vi "Configure Modulation (AM).vi"(4 "Modulation Waveform (0: Sine)":u16(ring) items=["Sine", "Square", "Triangle", "UpRamp", "DnRamp", "Noise", "Arb"], 5 "Channel (1:Channel 1)":i32(ring)=1 items=["Channel 1"=1, "Channel 2"=2], 6 "Modulation Frequency (100 Hz)":dbl=100.0, 7 "Enable Amplitude Modulation (T:Enable)":bool=TRUE, 8 "error in (no error)":errorcluster, 9 "Modulation Depth (0.0 %)":dbl min=0.0 max=120.0 format="%.1f", 10 "AM Source (0: Internal)":u16(ring) items=["Internal", "External"], 11 "VISA resource name":refnum<visa-resource-name>) -> (0 "error out":errorcluster, 3 "VISA resource name out":refnum<visa-resource-name>)   [LabVIEW 2015, in "SDG X Series.lvlib"]
doc: "Configures and enables amplitude modulation (AM). In AM, the amplitude of the carrier is varied by the amplitude of the modulating waveform. \n\n<B>Note:</B> The carrier waveform shape and parameters are set by the Configure Standard Waveform VI."
uses:
  <instrlib>/SDG X Series/SDG X Series.lvlib
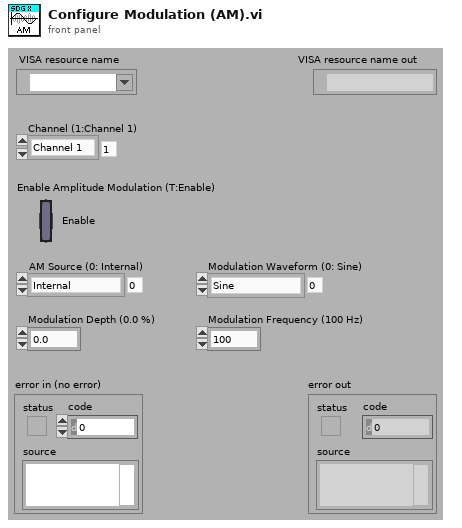
[diagram p1: front panel]
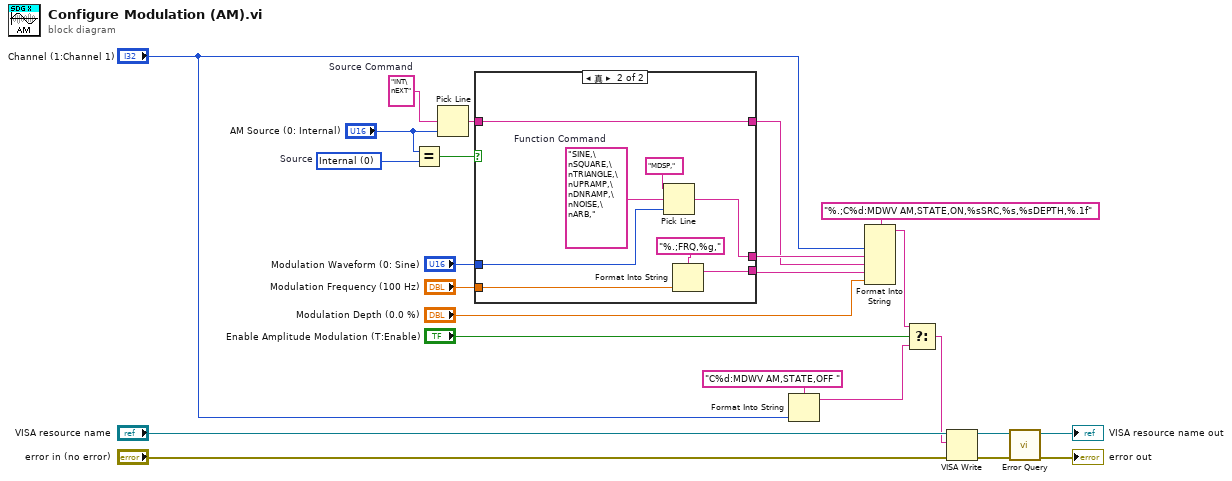
[diagram p0: block diagram]
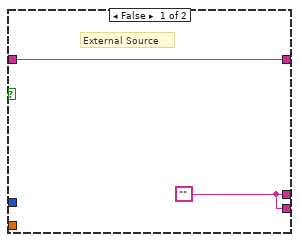
[diagram p2: hidden frame]
diagram:
  w18 = u16 0 items=["Internal", "External"]  # Source
  w19 = "INT\nEXT"  # Source Command
  n1 = Equal?(x="AM Source (0: Internal)", y=w18) -> (x = y?=w17:bool)
  n2 = Pick Line(multi-line string=w19, line index="AM Source (0: Internal)") -> (output string=w16:string)  [unwired: 1 in]
  n3 = case shown="真" w17 {
    tunnel: w16 -> [w26 w32]
    tunnel: "Modulation Waveform (0: Sine)" -> [_ w33]
    tunnel: "Modulation Frequency (100 Hz)" -> [_ w29]
    tunnel: [w26 w32] -> w13
    tunnel: [w25 w30] -> w14
    tunnel: [w25 w27] -> w12
    frame False {
      w25 = ""
      # "External Source"
    }
    frame True {
      w34 = "SINE,\nSQUARE,\nTRIANGLE,\nUPRAMP,\nDNRAMP,\nNOISE,\nARB,"  # Function Command
      n4 = Pick Line(string ("")="MDSP,", multi-line string=w34, line index=w33) -> (output string=w30:string)
      n5 = Format Into String(format string="%.;FRQ,%g,", w29) -> (resulting string=w27:string)  [unwired: 2 in, 1 out]
    }
  }
  n6 = Format Into String(format string="C%d:MDWV AM,STATE,OFF ", "Channel (1:Channel 1)") -> (resulting string=w6:string)  [unwired: 2 in, 1 out]
  n7 = Format Into String(format string="%.;C%d:MDWV AM,STATE,ON,%sSRC,%s,%sDEPTH,%.1f", "Channel (1:Channel 1)", w14, w13, w12, "Modulation Depth (0.0 %)") -> (resulting string=w9:string)  [unwired: 2 in, 1 out]
  n8 = Select(t=w9, s="Enable Amplitude Modulation (T:Enable)", f=w6) -> (s? t:f=w8:string)
  n9 = VISA Write(VISA resource name="VISA resource name", write buffer=w8, error in (no error)="error in (no error)") -> (VISA resource name out=w2:refnum<visa-resource-name>, error out=w1:errorcluster)  [unwired: 1 out]
  n10 = call <instrlib>:"Error Query.vi"("error in (no error)"=w1, "VISA resource name"=w2) -> ("error out"=→"error out":errorcluster, "VISA resource name out"=→"VISA resource name out":refnum<visa-resource-name>)  [unwired: 6 in, 2 out]
